vi "Calculator.vi"() -> ()   [LabVIEW 2022 SP3]
uses:
  <vilib>/gmath/NI_Gmath.lvlib
panel:
  in  "%":bool
  in  "pi":bool
  in  "^":bool
  in  "^2":bool
  in  "InputToM1":bool=TRUE
  out "M2":string
  out "M1":string
  in  "M+":bool
  in  "M-":bool
  in  "MR":bool
  in  "MC":bool
  in  "CE":bool
  in  "+/-":bool
  out "Using Time (sec)":dbl
  out "Current Time":timestamp format="%<%Y/%m/%d %H:%M:%S>T"
  in  "power":bool
  out "main":string
  in  "Off":bool
  in  "backspace":bool
  in  "(":bool
  in  ")":bool
  in  "C":bool
  in  "1/x":bool
  in  "Sqrt":bool
  in  "=":bool
  in  "+":bool
  in  "-":bool
  in  "*":bool
  in  "/":bool
  in  "7":bool
  in  "8":bool
  in  "9":bool
  in  "6":bool
  in  "5":bool
  in  "4":bool
  in  "1":bool
  in  "2":bool
  in  "3":bool
  in  ".":bool
  in  "0":bool
  in  "Error":bool
  in  "last_op":u32
  in  "if M":bool
  out "timer_i":dbl
  out "positive":bool=TRUE
  out "answer":dbl
  in  "if\"=\"":bool
  # "Student ID: 111550073"
  # "Guide book:\n\nC : The memories and the screen will be cleared up.\nCE : Only the screen will be cleared up.\n<- : Backspace.\n\n+, -, *, / : When the answer is displayed, you can press then to keep calculate.\n\n1/x : When the string ends with a number, \n         it will input \"(1/\" before the number and a \")\" must be input after you finish inputting.\n         When it ends with an operation symbol, \n         it will input \"(1/\", and a \")\" must be input after you finish inputting.\n         When answer is displayed and it is pressed, you won't have to input a \")\".\n^: Power of. It will input \"^\".\nsqare: It will input \"^2\"\nsqrt : Sqareroot.\n      When the string ends with a number, \n      it will input \"sqrt(\" before the number and a \")\" must be input after you finish inputting.\n      When it ends with an operation symbol, \n      it will input \"sqrt(\", and a \")\" must be input after you finish inputting.\n      When answer is displayed and it is pressed, you won't have to input a \")\".\n£k : pi(x).\n      When the string ends with a number, \n      it will input \"pi(\" before the number and a \")\" must be input after you finish inputting.\n      When it ends with an operation symbol, \n      it will input \"pi(\", and a \")\" must be input after you finish inputting.\n      When answer is displayed and it is pressed, you won't have to input a \")\".\n%: It will input \"*0.01\".\n      When the answer is displayed, you can press then to keep calculate.\n\n+/- : When pressed, it will input a negative symbol before the last number you input.\n          If clicked second time, it will remove the negative symbol.\n          p.s. When the operation symbol is \"-\", it won't change it into a \"+\".\n\nM+, M- : The value on the screen or the answer of the formula will be stored. \nMR : The value which is stored into memory will display on the screen.\nMC : The value in memory will be cleared up. (Either memory 1 or memory 2) \n\nUsing M1& M2: When vertical switch is up, the value will stored into M1; \n                              otherwise, it will be stored into M2."
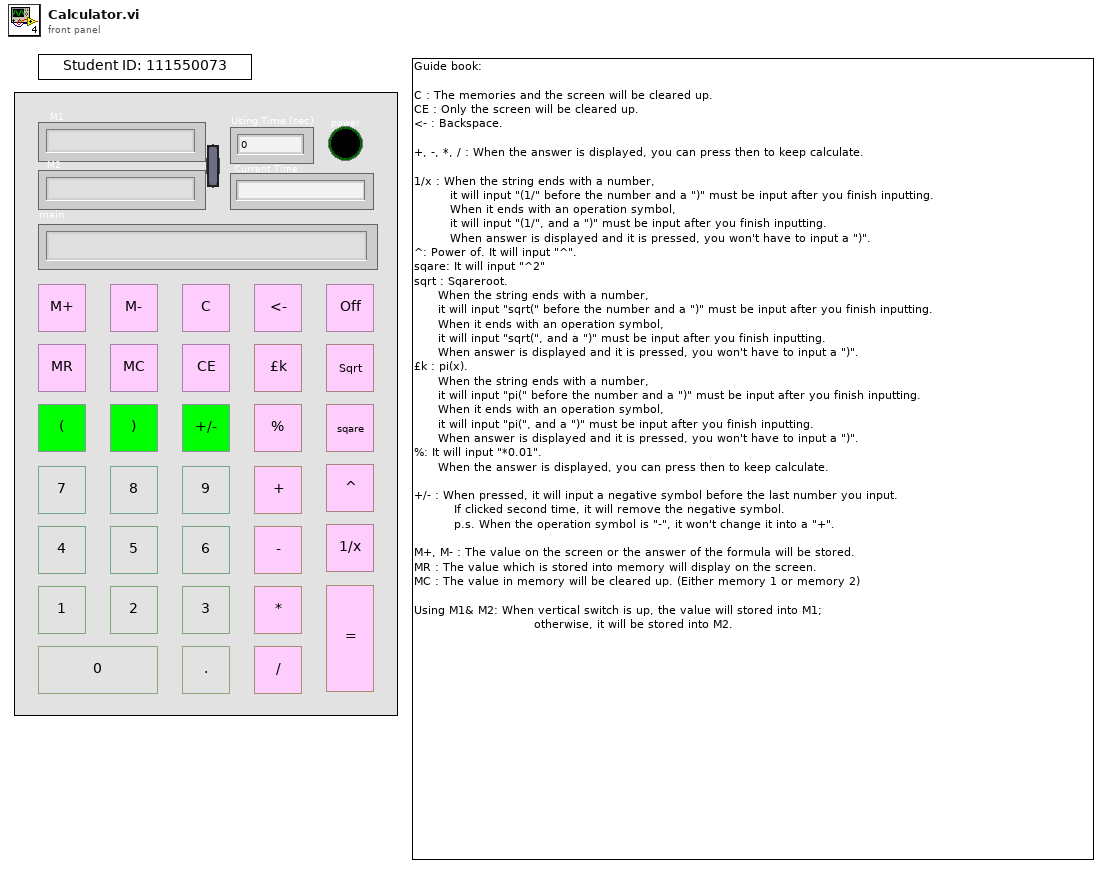
[diagram p1: front panel]
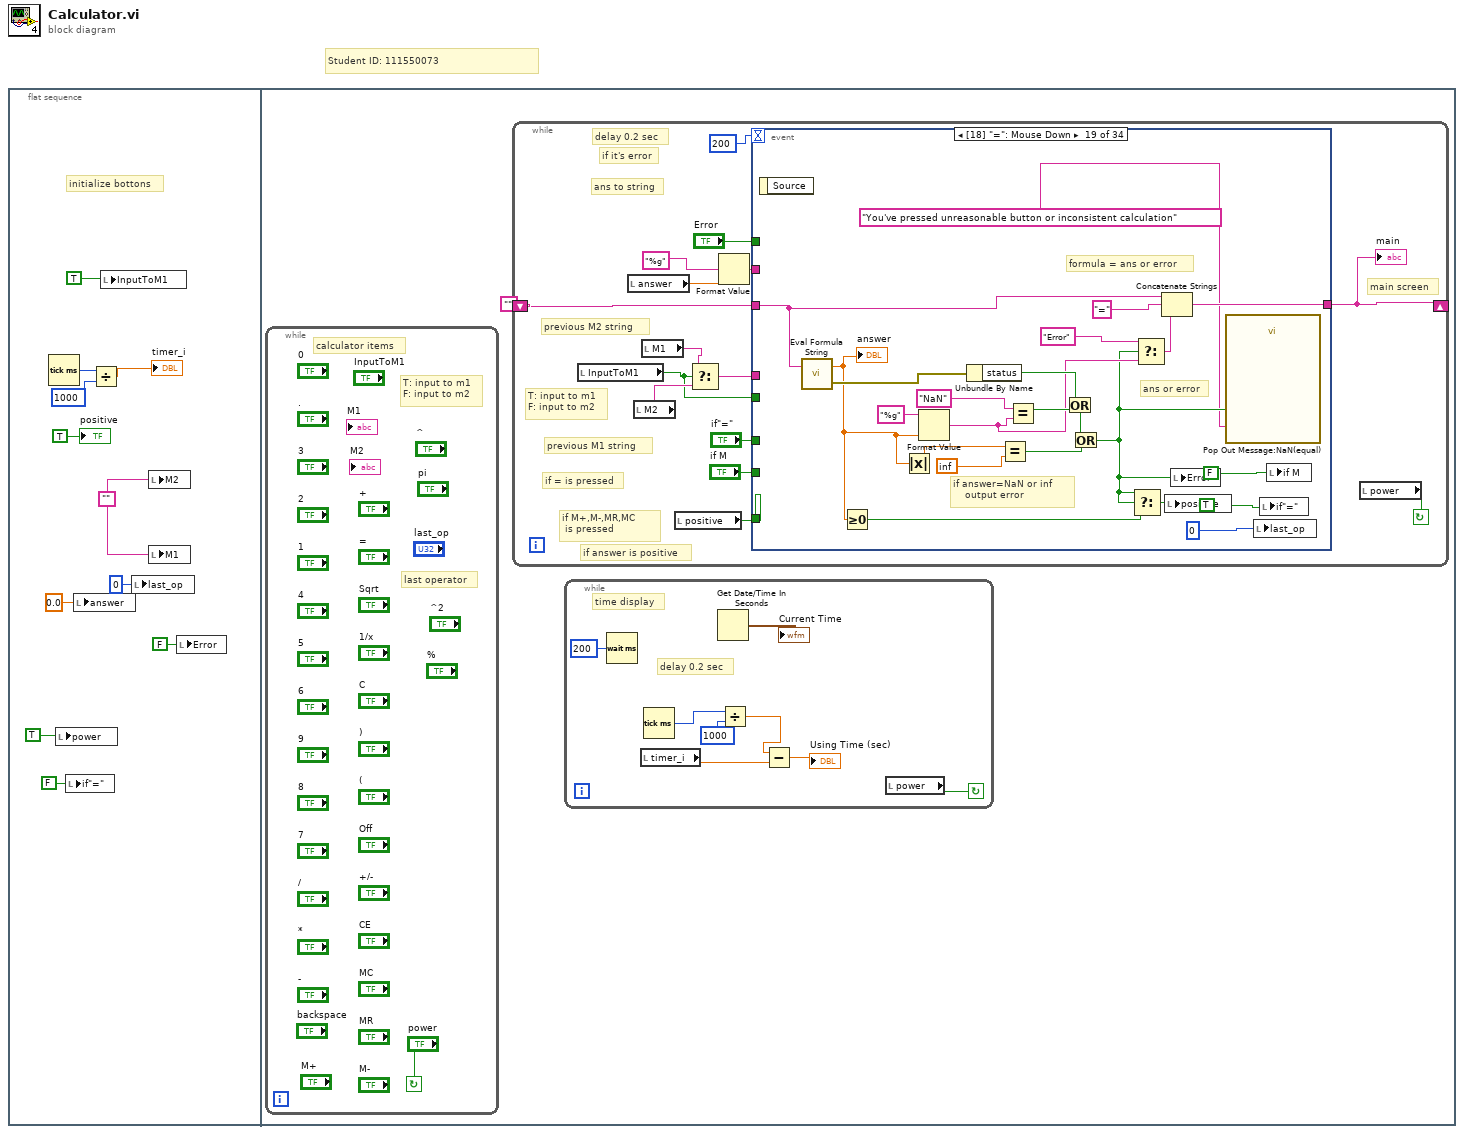
[diagram p0: block diagram]
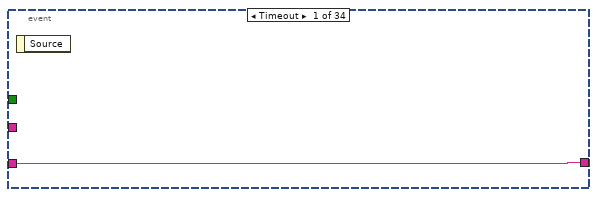
[diagram p2: hidden frame]
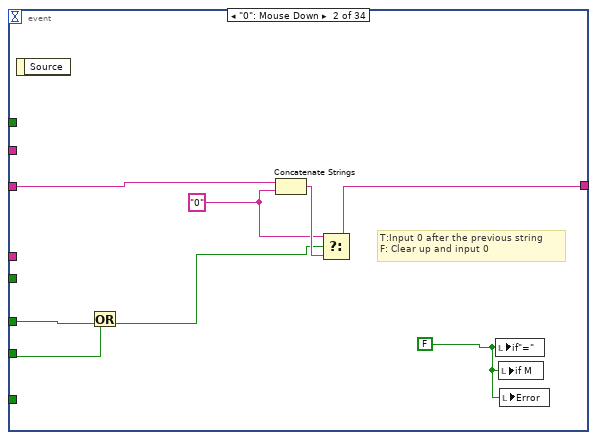
[diagram p3: hidden frame]
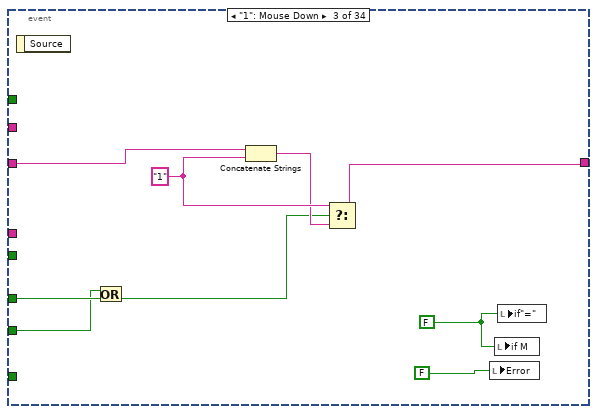
[diagram p4: hidden frame]
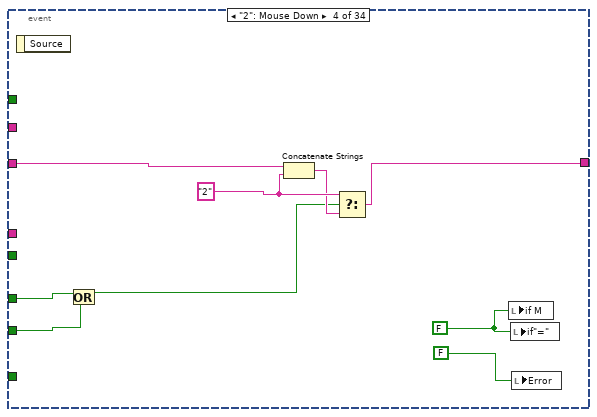
[diagram p5: hidden frame]
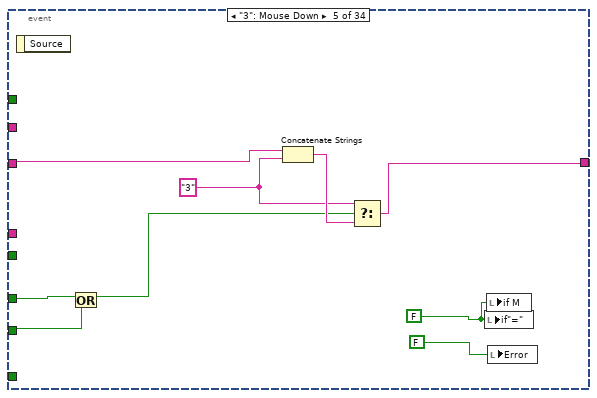
[diagram p6: hidden frame]
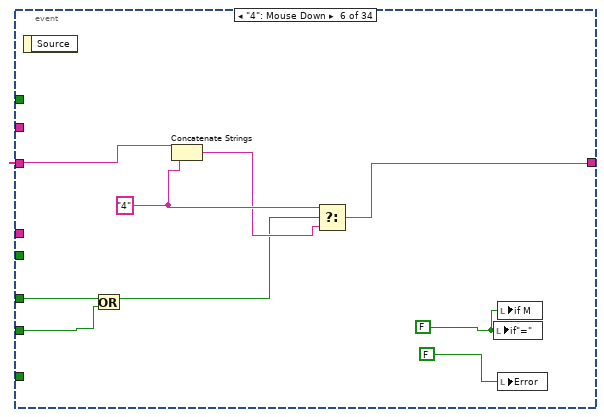
[diagram p7: hidden frame]
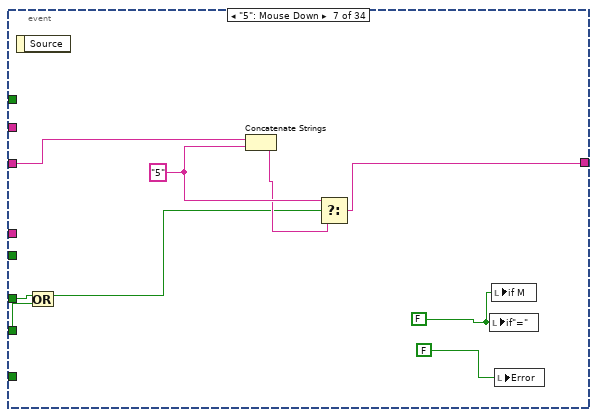
[diagram p8: hidden frame]
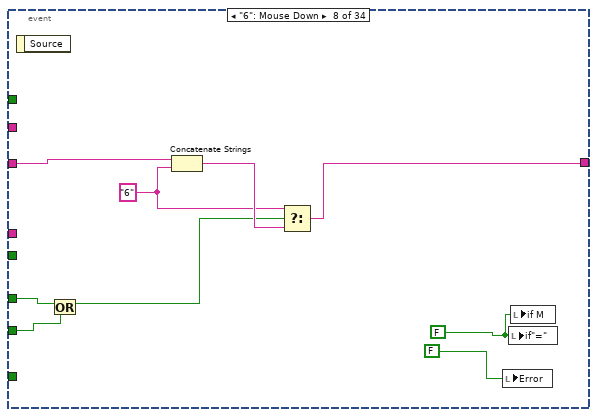
[diagram p9: hidden frame]
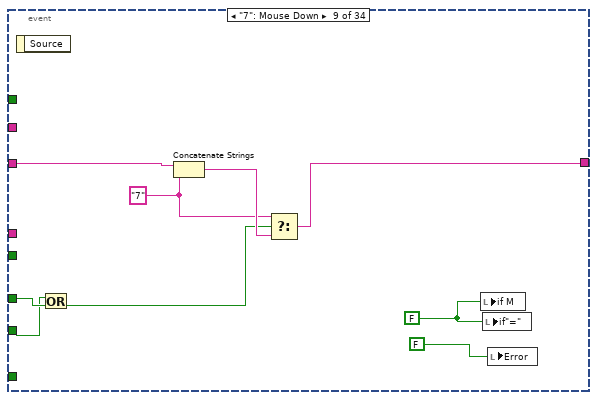
[diagram p10: hidden frame]
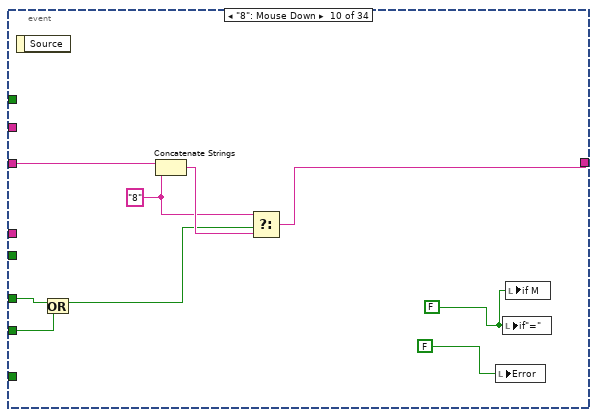
[diagram p11: hidden frame]
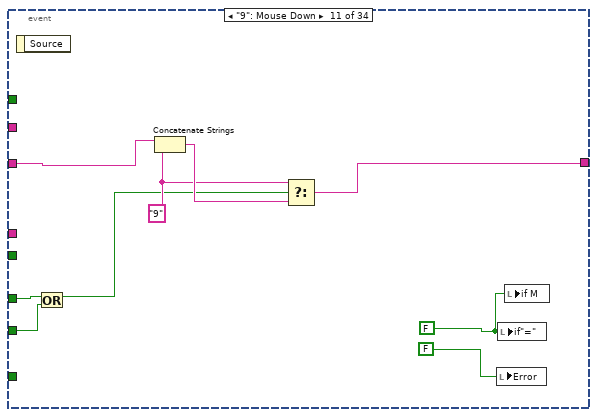
[diagram p12: hidden frame]
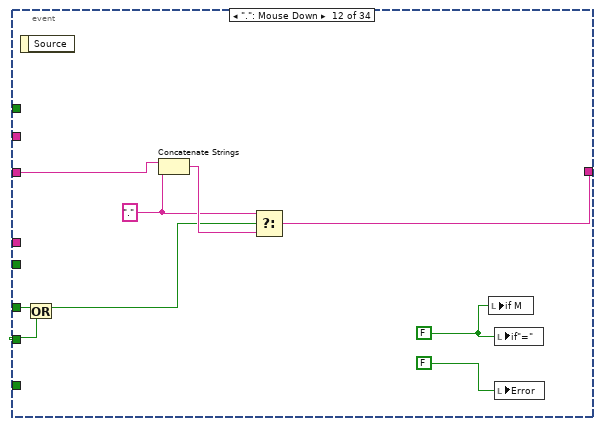
[diagram p13: hidden frame]
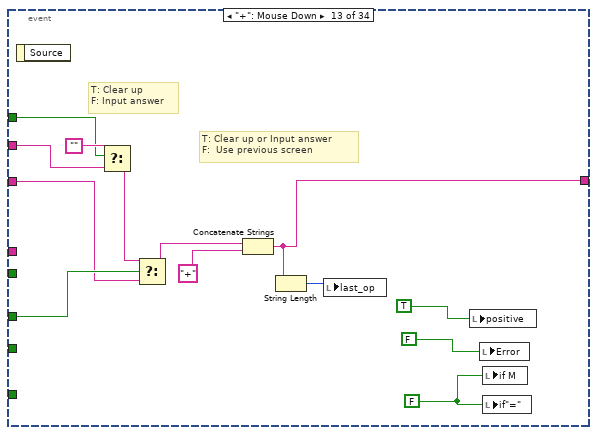
[diagram p14: hidden frame]
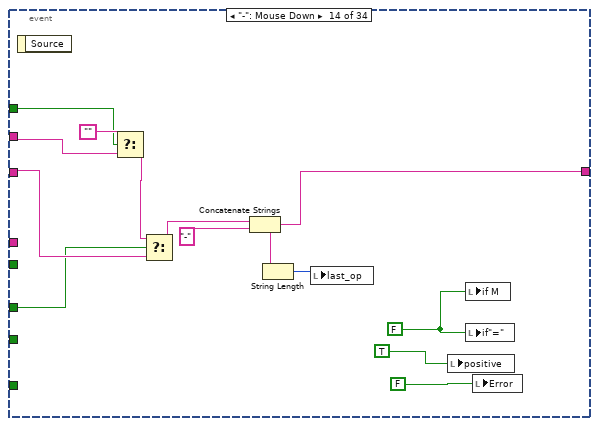
[diagram p15: hidden frame]
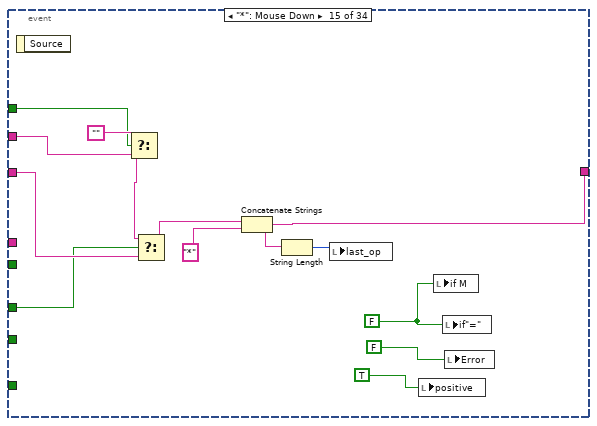
[diagram p16: hidden frame]
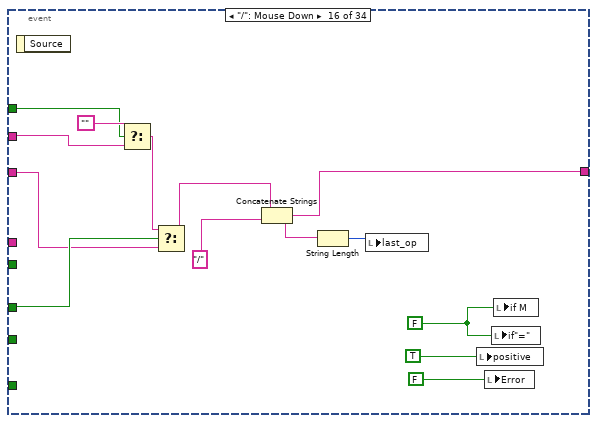
[diagram p17: hidden frame]
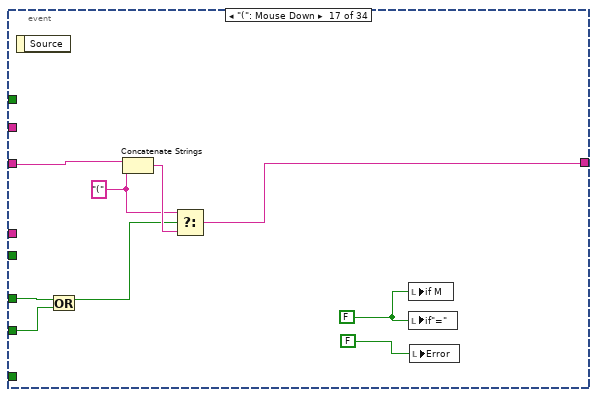
[diagram p18: hidden frame]
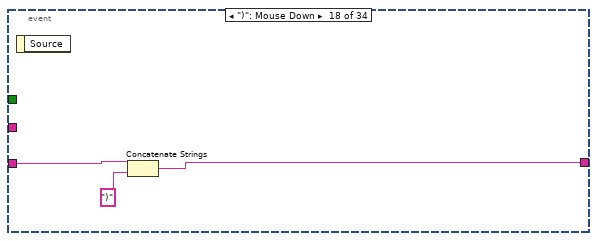
[diagram p19: hidden frame]
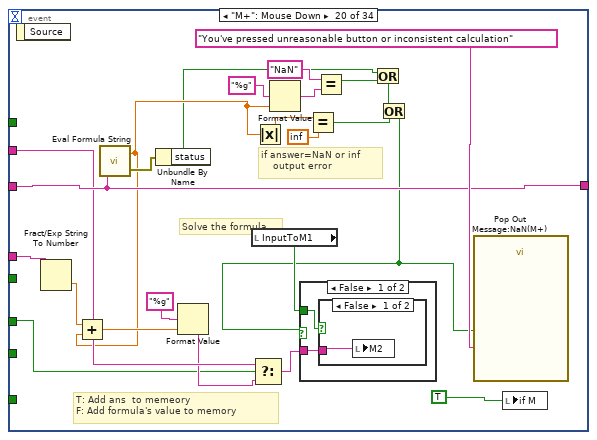
[diagram p20: hidden frame]
diagram:
  # "Student ID: 111550073"
  n1 = flat-sequence {
    frame #0 {
      w3 = ""
      # "initialize bottons"
      n2 = Tick Count (ms)() -> (millisecond timer value=w6:u32)
      n3 = local write "power"(TRUE ("stop")) -> ()
      n4 = local write "if\"=\""(FALSE ("if\"=\"")) -> ()
      n5 = local write "answer"(0.0 ("pre_ans")) -> ()
      n6 = Divide(x=w6, y=u32 1000) -> (x/y=→"timer_i":dbl)
      n7 = local write "InputToM1"(TRUE) -> ()
      n8 = local write "last_op"(u32 0 ("last_op")) -> ()
      n9 = local write "M2"(w3) -> ()
      n10 = local write "M1"(w3) -> ()
      n11 = local write "Error"(FALSE ("Error")) -> ()
      "positive" <- TRUE ("Boolean")
    }
    frame #1 {
      n12 = while {
        stop <- "power" continue-if-true
        # "last operator"
        # "T: input to m1\nF: input to m2"
        # "calculator items"
      }
      n13 = while {
        shift-right: [w33] -> _
        shift-left: "" -> [w21]
        stop <- w24 continue-if-true
        # "delay 0.2 sec"
        # "if it's error"
        # "main screen"
        # "if M+,M-,MR,MC\n is pressed"
        # "if = is pressed"
        # "previous M2 string"
        # "previous M1 string"
        # "T: input to m1\nF: input to m2"
        # "if answer is positive"
        # "ans to string"
        n14 = local read "InputToM1"() -> (w23:bool)
        n15 = local read "answer"() -> (w31:dbl)
        n16 = local read "M2"() -> (w27:string)
        n17 = local read "M1"() -> (w26:string)
        n18 = local read "positive"() -> (w29:bool)
        n19 = Select(t=w26, s=w23, f=w27) -> (s? t:f=w25:string)
        n20 = Format Value(format string="%g", value (0)=w31) -> (output string=w30:string)  [unwired: 1 in]
        n21 = event shown="[18] \"=\": Mouse Down" {
          selector: _ -> [_ _ _ _ _ _ _ _ _ _ _ _ _ _ _ _ _ _ _ _ _ _ _ _ _ _ _ _ _ _ _ _ _ _]
          dyn-events: _ -> [_ _ _ _ _ _ _ _ _ _ _ _ _ _ _ _ _ _ _ _ _ _ _ _ _ _ _ _ _ _ _ _ _ _]
          timeout: 200 -> [_ _ _ _ _ _ _ _ _ _ _ _ _ _ _ _ _ _ _ _ _ _ _ _ _ _ _ _ _ _ _ _ _ _]
          tunnel: [w36 w41 w50 w59 w67 w78 w85 w94 w103 w112 w118 w130 w141 w156 w168 w180 w191 w196 w213 w237 w266 w283 w294 w304 w309 w323 w339 w346 w352 w365 w379 w391 w405 w419] -> w33
          tunnel: w21 -> [w36 w44 w53 w62 w71 w80 w89 w98 w105 w113 w122 w131 w145 w159 w172 w185 w192 w198 w218 w237 w266 w282 w294 w305 w313 w322 w342 w343 w354 w366 w381 w394 w417 w422]
          tunnel: "if\"=\"" -> [_ w42 w51 w60 w68 w79 w86 w95 w104 w114 w123 w132 w146 w149 w162 w186 w193 _ _ w233 w263 w284 _ _ _ w321 _ _ w353 w364 w378 w395 w409 w424]
          tunnel: w29 -> [_ _ _ _ _ _ _ _ _ _ _ _ _ _ _ _ _ _ _ _ _ _ _ _ _ w324 _ _ _ _ _ _ _ _]
          tunnel: w30 -> [_ _ _ _ _ _ _ _ _ _ _ _ w138 w152 w164 w176 _ _ _ w236 w264 _ _ _ _ w315 _ _ w355 w367 w380 w396 w412 w423]
          tunnel: "if M" -> [_ w39 w47 w56 w65 w74 w83 w92 w101 w110 w120 w128 _ _ _ _ w189 _ _ _ _ _ _ _ _ _ _ _ _ _ _ _ _ _]
          tunnel: w25 -> [_ _ _ _ _ _ _ _ _ _ _ _ _ _ _ _ _ _ _ w243 w274 w281 _ _ _ _ _ _ _ _ _ _ _ _]
          tunnel: w23 -> [_ _ _ _ _ _ _ _ _ _ _ _ _ _ _ _ _ _ _ _ _ _ w288 _ _ _ _ _ _ _ _ _ _ _]
          tunnel: "Error" -> [_ _ _ _ _ _ _ _ _ _ _ _ w135 w148 w161 w174 _ _ _ _ _ _ _ _ _ w314 _ _ w349 w368 w382 w397 w406 _]
          event Timeout {
            n22 = event-data() -> ()  [unwired: 1 in, 1 out]
          }
          event "0": Mouse Down {
            w38 = FALSE ("if\"=\"")
            w37 = "0"
            # "T:Input 0 after the previous string\nF: Clear up and input 0"
            n23 = event-data() -> ()  [unwired: 1 in, 1 out]
            n24 = Or(x=w39, y=w42) -> (x .or. y?=w40:bool)
            n25 = Concatenate Strings(w44, w37) -> (w43:string)
            n26 = Select(t=w37, s=w40, f=w43) -> (s? t:f=w41:string)
            n27 = local write "if\"=\""(w38) -> ()
            n28 = local write "if M"(w38) -> ()
            n29 = local write "Error"(w38) -> ()
          }
          event "1": Mouse Down {
            w46 = FALSE ("if\"=\"")
            w52 = "1"
            n30 = event-data() -> ()  [unwired: 1 in, 1 out]
            n31 = Or(x=w47, y=w51) -> (x .or. y?=w48:bool)
            n32 = Concatenate Strings(w53, w52) -> (w49:string)
            n33 = Select(t=w52, s=w48, f=w49) -> (s? t:f=w50:string)
            n34 = local write "Error"(FALSE ("Error")) -> ()
            n35 = local write "if M"(w46) -> ()
            n36 = local write "if\"=\""(w46) -> ()
          }
          event "2": Mouse Down {
            w55 = FALSE ("if\"=\"")
            w61 = "2"
            n37 = event-data() -> ()  [unwired: 1 in, 1 out]
            n38 = Or(x=w60, y=w56) -> (x .or. y?=w57:bool)
            n39 = Concatenate Strings(w62, w61) -> (w58:string)
            n40 = Select(t=w61, s=w57, f=w58) -> (s? t:f=w59:string)
            n41 = local write "if M"(w55) -> ()
            n42 = local write "if\"=\""(w55) -> ()
            n43 = local write "Error"(FALSE ("Error")) -> ()
          }
          event "3": Mouse Down {
            w64 = FALSE ("if\"=\"")
            w69 = "3"
            n44 = event-data() -> ()  [unwired: 1 in, 1 out]
            n45 = Or(x=w68, y=w65) -> (x .or. y?=w66:bool)
            n46 = Concatenate Strings(w71, w69) -> (w70:string)
            n47 = Select(t=w69, s=w66, f=w70) -> (s? t:f=w67:string)
            n48 = local write "if\"=\""(w64) -> ()
            n49 = local write "if M"(w64) -> ()
            n50 = local write "Error"(FALSE ("Error")) -> ()
          }
          event "4": Mouse Down {
            w73 = FALSE ("if\"=\"")
            w77 = "4"
            n51 = event-data() -> ()  [unwired: 1 in, 1 out]
            n52 = Or(x=w79, y=w74) -> (x .or. y?=w75:bool)
            n53 = Concatenate Strings(w80, w77) -> (w76:string)
            n54 = Select(t=w77, s=w75, f=w76) -> (s? t:f=w78:string)
            n55 = local write "if\"=\""(w73) -> ()
            n56 = local write "if M"(w73) -> ()
            n57 = local write "Error"(FALSE ("Error")) -> ()
          }
          event "5": Mouse Down {
            w82 = FALSE ("if\"=\"")
            w88 = "5"
            n58 = event-data() -> ()  [unwired: 1 in, 1 out]
            n59 = Or(x=w86, y=w83) -> (x .or. y?=w84:bool)
            n60 = Concatenate Strings(w89, w88) -> (w87:string)
            n61 = Select(t=w88, s=w84, f=w87) -> (s? t:f=w85:string)
            n62 = local write "if\"=\""(w82) -> ()
            n63 = local write "if M"(w82) -> ()
            n64 = local write "Error"(FALSE ("Error")) -> ()
          }
          event "6": Mouse Down {
            w91 = FALSE ("if\"=\"")
            w96 = "6"
            n65 = event-data() -> ()  [unwired: 1 in, 1 out]
            n66 = Or(x=w95, y=w92) -> (x .or. y?=w93:bool)
            n67 = Concatenate Strings(w98, w96) -> (w97:string)
            n68 = Select(t=w96, s=w93, f=w97) -> (s? t:f=w94:string)
            n69 = local write "Error"(FALSE ("Error")) -> ()
            n70 = local write "if\"=\""(w91) -> ()
            n71 = local write "if M"(w91) -> ()
          }
          event "7": Mouse Down {
            w100 = FALSE ("if\"=\"")
            w106 = "7"
            n72 = event-data() -> ()  [unwired: 1 in, 1 out]
            n73 = Or(x=w101, y=w104) -> (x .or. y?=w102:bool)
            n74 = Concatenate Strings(w105, w106) -> (w107:string)
            n75 = Select(t=w106, s=w102, f=w107) -> (s? t:f=w103:string)
            n76 = local write "if M"(w100) -> ()
            n77 = local write "if\"=\""(w100) -> ()
            n78 = local write "Error"(FALSE ("Error")) -> ()
          }
          event "8": Mouse Down {
            w109 = FALSE ("if\"=\"")
            w115 = "8"
            n79 = event-data() -> ()  [unwired: 1 in, 1 out]
            n80 = Or(x=w114, y=w110) -> (x .or. y?=w111:bool)
            n81 = Concatenate Strings(w113, w115) -> (w116:string)
            n82 = Select(t=w115, s=w111, f=w116) -> (s? t:f=w112:string)
            n83 = local write "Error"(FALSE ("Error")) -> ()
            n84 = local write "if\"=\""(w109) -> ()
            n85 = local write "if M"(w109) -> ()
          }
          event "9": Mouse Down {
            w119 = FALSE ("if\"=\"")
            w124 = "9"
            n86 = event-data() -> ()  [unwired: 1 in, 1 out]
            n87 = Or(x=w123, y=w120) -> (x .or. y?=w121:bool)
            n88 = Concatenate Strings(w122, w124) -> (w125:string)
            n89 = Select(t=w124, s=w121, f=w125) -> (s? t:f=w118:string)
            n90 = local write "Error"(FALSE ("Error")) -> ()
            n91 = local write "if\"=\""(w119) -> ()
            n92 = local write "if M"(w119) -> ()
          }
          event ".": Mouse Down {
            w127 = FALSE ("if\"=\"")
            w133 = "."
            n93 = event-data() -> ()  [unwired: 1 in, 1 out]
            n94 = Or(x=w132, y=w128) -> (x .or. y?=w129:bool)
            n95 = Concatenate Strings(w131, w133) -> (w134:string)
            n96 = Select(t=w133, s=w129, f=w134) -> (s? t:f=w130:string)
            n97 = local write "if M"(w127) -> ()
            n98 = local write "if\"=\""(w127) -> ()
            n99 = local write "Error"(FALSE ("Error")) -> ()
          }
          event "+": Mouse Down {
            w144 = FALSE ("if\"=\"")
            # "T: Clear up or Input answer  \nF:  Use previous screen"
            # "T: Clear up\nF: Input answer"
            n100 = event-data() -> ()  [unwired: 1 in, 1 out]
            n101 = Select(t="", s=w135, f=w138) -> (s? t:f=w139:string)
            n102 = Select(t=w139, s=w146, f=w145) -> (s? t:f=w147:string)
            n103 = Concatenate Strings(w147, "+") -> (w141:string)
            n104 = String Length(string=w141) -> (length=w142:i32)
            n105 = local write "last_op"(w142) -> ()
            n106 = local write "positive"(TRUE ("positive")) -> ()
            n107 = local write "Error"(FALSE ("Error")) -> ()
            n108 = local write "if M"(w144) -> ()
            n109 = local write "if\"=\""(w144) -> ()
          }
          event "-": Mouse Down {
            w158 = FALSE ("if\"=\"")
            n110 = event-data() -> ()  [unwired: 1 in, 1 out]
            n111 = Select(t="", s=w148, f=w152) -> (s? t:f=w151:string)
            n112 = Select(t=w151, s=w149, f=w159) -> (s? t:f=w160:string)
            n113 = Concatenate Strings(w160, "-") -> (w156:string)
            n114 = String Length(string=w156) -> (length=w155:i32)
            n115 = local write "last_op"(w155) -> ()
            n116 = local write "positive"(TRUE ("positive")) -> ()
            n117 = local write "if M"(w158) -> ()
            n118 = local write "if\"=\""(w158) -> ()
            n119 = local write "Error"(FALSE ("Error")) -> ()
          }
          event "*": Mouse Down {
            w171 = FALSE ("if\"=\"")
            n120 = event-data() -> ()  [unwired: 1 in, 1 out]
            n121 = Select(t="", s=w161, f=w164) -> (s? t:f=w163:string)
            n122 = Select(t=w163, s=w162, f=w172) -> (s? t:f=w173:string)
            n123 = Concatenate Strings(w173, "*") -> (w168:string)
            n124 = String Length(string=w168) -> (length=w169:i32)
            n125 = local write "last_op"(w169) -> ()
            n126 = local write "positive"(TRUE ("positive")) -> ()
            n127 = local write "if M"(w171) -> ()
            n128 = local write "if\"=\""(w171) -> ()
            n129 = local write "Error"(FALSE ("Error")) -> ()
          }
          event "/": Mouse Down {
            w183 = FALSE ("if\"=\"")
            n130 = event-data() -> ()  [unwired: 1 in, 1 out]
            n131 = Select(t="", s=w174, f=w176) -> (s? t:f=w175:string)
            n132 = Select(t=w175, s=w186, f=w185) -> (s? t:f=w184:string)
            n133 = Concatenate Strings(w184, "/") -> (w180:string)
            n134 = String Length(string=w180) -> (length=w181:i32)
            n135 = local write "last_op"(w181) -> ()
            n136 = local write "positive"(TRUE ("positive")) -> ()
            n137 = local write "Error"(FALSE ("Error")) -> ()
            n138 = local write "if\"=\""(w183) -> ()
            n139 = local write "if M"(w183) -> ()
          }
          event "(": Mouse Down {
            w188 = FALSE ("if\"=\"")
            w194 = "("
            n140 = event-data() -> ()  [unwired: 1 in, 1 out]
            n141 = Or(x=w193, y=w189) -> (x .or. y?=w190:bool)
            n142 = Concatenate Strings(w192, w194) -> (w195:string)
            n143 = Select(t=w194, s=w190, f=w195) -> (s? t:f=w191:string)
            n144 = local write "if M"(w188) -> ()
            n145 = local write "if\"=\""(w188) -> ()
            n146 = local write "Error"(FALSE ("Error")) -> ()
          }
          event ")": Mouse Down {
            n147 = event-data() -> ()  [unwired: 1 in, 1 out]
            n148 = Concatenate Strings(w198, ")") -> (w196:string)
          }
          event "=": Mouse Down {
            # "if answer=NaN or inf \n    output error"
            # "ans or error"
            # "formula = ans or error"
            n149 = event-data() -> ()  [unwired: 1 in, 1 out]
            n150 = call <vilib>:"Eval Formula String.vi"("formula"=w218) -> ("error out"=w216:errorcluster, "y value"=w199:dbl)  [unwired: 1 in]
            "answer" <- w199
            n151 = Greater Or Equal To 0?(x=w199) -> (x >= 0?=w204:bool)
            n152 = Absolute Value(x=w199) -> (abs(x)=w212:dbl)
            n153 = Format Value(format string="%g", value (0)=w199) -> (output string=w205:string)  [unwired: 1 in]
            n154 = Unbundle By Name(w216) -> ("status"=w208:bool)
            n155 = Equal?(x=w212, y=inf) -> (x = y?=w210:bool)
            n156 = Equal?(x="NaN", y=w205) -> (x = y?=w206:bool)
            n157 = Or(x=w208, y=w206) -> (x .or. y?=w207:bool)
            n158 = Or(x=w207, y=w210) -> (x .or. y?=w201:bool)
            n159 = Select(t=w201, s=w201, f=w204) -> (s? t:f=w203:bool)
            n160 = Select(t="Error" ("f"), s=w201, f=w205) -> (s? t:f=w214:string)
            n161 = Concatenate Strings(w218, "=" ("string"), w214) -> (w213:string)
            n162 = local write "positive"(w203) -> ()
            n163 = local write "Error"(w201) -> ()
            n164 = call "Pop Out Message:NaN(equal)"("Enable"=w201, "Message"="You've pressed unreasonable button or inconsistent calculation") -> ()  [unwired: 8 in, 2 out]
            n165 = local write "last_op"(u32 0 ("last_op")) -> ()
            n166 = local write "if\"=\""(TRUE ("if\"=\"")) -> ()
            n167 = local write "if M"(FALSE ("if\"=\"")) -> ()
          }
          event "M+": Mouse Down {
            # "if answer=NaN or inf \n    output error"
            # "Solve the formula"
            # "T: Add ans  to memeory\nF: Add formula's value to memory"
            n168 = event-data() -> ()  [unwired: 1 in, 1 out]
            n169 = Fract/Exp String To Number(string=w243) -> (number=w242:dbl)  [unwired: 3 in, 1 out]
            n170 = call <vilib>:"Eval Formula String.vi"("formula"=w237) -> ("error out"=w239:errorcluster, "y value"=w224:dbl)  [unwired: 1 in]
            n171 = Add(x=w242, y=w224) -> (x+y=w244:dbl)
            n172 = Unbundle By Name(w239) -> ("status"=w223:bool)
            n173 = Format Value(format string="%g", value (0)=w244) -> (output string=w235:string)  [unwired: 1 in]
            n174 = local read "InputToM1"() -> (w238:bool)
            n175 = Select(t=w236, s=w233, f=w235) -> (s? t:f=w234:string)
            n176 = Absolute Value(x=w224) -> (abs(x)=w232:dbl)
            n177 = Format Value(format string="%g", value (0)=w224) -> (output string=w228:string)  [unwired: 1 in]
            n178 = Equal?(x=w232, y=inf) -> (x = y?=w231:bool)
            n179 = Equal?(x="NaN", y=w228) -> (x = y?=w229:bool)
            n180 = Or(x=w223, y=w229) -> (x .or. y?=w230:bool)
            n181 = Or(x=w230, y=w231) -> (x .or. y?=w222:bool)
            n182 = case shown="False" w222 {
              tunnel: w238 -> [w247 _]
              tunnel: w234 -> [w246 _]
              frame False {
                n183 = case shown="False" w247 {
                  tunnel: w246 -> [w248 w249]
                  frame False {
                    n184 = local write "M2"(w248) -> ()
                  }
                  frame True {
                    n185 = local write "M1"(w249) -> ()
                  }
                }
              }
              frame True {
              }
            }
            n186 = call "Pop Out Message:NaN(M+)"("Enable"=w222, "Message"="You've pressed unreasonable button or inconsistent calculation") -> ()  [unwired: 8 in, 2 out]
            n187 = local write "if M"(TRUE ("if\"=\"")) -> ()
          }
          event "M-": Mouse Down {
            # "if answer=NaN or inf \n    output error"
            # "string to float"
            # "T: Add  negative ans  to memeory\nF: Add formula's negative value to     memory"
            n188 = event-data() -> ()  [unwired: 1 in, 1 out]
            n189 = call <vilib>:"Eval Formula String.vi"("formula"=w266) -> ("error out"=w271:errorcluster, "y value"=w252:dbl)  [unwired: 1 in]
            n190 = Fract/Exp String To Number(string=w274) -> (number=w273:dbl)  [unwired: 3 in, 1 out]
            n191 = Unbundle By Name(w271) -> ("status"=w251:bool)
            n192 = Absolute Value(x=w252) -> (abs(x)=w256:dbl)
            n193 = Format Value(format string="%g", value (0)=w252) -> (output string=w260:string)  [unwired: 1 in]
            n194 = Equal?(x=w256, y=inf) -> (x = y?=w257:bool)
            n195 = Equal?(x="NaN", y=w260) -> (x = y?=w259:bool)
            n196 = Or(x=w251, y=w259) -> (x .or. y?=w258:bool)
            n197 = Or(x=w258, y=w257) -> (x .or. y?=w250:bool)
            n198 = Select(t=0.0, s=w250, f=w252) -> (s? t:f=w268:dbl)
            n199 = Negate(x=w268) -> (-x=w276:dbl)
            n200 = Add(x=w273, y=w276) -> (x+y=w261:dbl)
            n201 = Format Value(format string="%g", value (0)=w261) -> (output string=w265:string)  [unwired: 1 in]
            n202 = Select(t=w264, s=w263, f=w265) -> (s? t:f=w262:string)
            n203 = local read "InputToM1"() -> (w267:bool)
            n204 = case shown="False" w250 {
              tunnel: w267 -> [w278 _]
              tunnel: w262 -> [w277 _]
              frame False {
                n205 = case shown="False" w278 {
                  tunnel: w277 -> [w279 w280]
                  frame False {
                    n206 = local write "M2"(w279) -> ()
                  }
                  frame True {
                    n207 = local write "M1"(w280) -> ()
                  }
                }
              }
              frame True {
              }
            }
            n208 = call "Display Message to User3"("Enable"=w250, "Message"="You've pressed unreasonable button or inconsistent calculation") -> ()  [unwired: 8 in, 2 out]
            n209 = local write "if M"(TRUE ("if\"=\"")) -> ()
          }
          event "MR": Mouse Down {
            # "T:Input memory after the previous string\nF: Clear up and input memory"
            n210 = event-data() -> ()  [unwired: 1 in, 1 out]
            n211 = Concatenate Strings(w282, w281) -> (w285:string)
            n212 = Select(t=w281, s=w284, f=w285) -> (s? t:f=w283:string)
            n213 = local write "if M"(TRUE ("if\"=\"")) -> ()
          }
          event "MC": Mouse Down {
            n214 = event-data() -> ()  [unwired: 1 in, 1 out]
            n215 = Select(t="2?", s=w288, f="1?" ("Message")) -> (s? t:f=w290:string)
            n216 = Concatenate Strings("Are you sure to clear up M" ("Message"), w290) -> (w292:string)
            n217 = call "Pop Out Message:MC"("Message"=w292) -> ("Yes"=w293:bool)  [unwired: 9 in, 1 out]
            n218 = case shown="True" w293 {
              frame False {
              }
              frame True {
                n219 = local read "InputToM1"() -> (w296:bool)
                n220 = case shown="False" w296 {
                  tunnel: "" -> [w297 w298]
                  frame False {
                    n221 = local write "M2"(w297) -> ()
                  }
                  frame True {
                    n222 = local write "M1"(w298) -> ()
                  }
                }
              }
            }
          }
          event "C": Mouse Down {
            n223 = event-data() -> ()  [unwired: 1 in, 1 out]
            n224 = Concatenate Strings("Are you sure to clear up " ("Message"), "the screen and memory?" ("string")) -> (w301:string)
            n225 = call "Pop Out Message:C"("Message"=w301) -> ("Yes"=w300:bool)  [unwired: 9 in, 1 out]
            n226 = case shown="True" w300 {
              frame False {
              }
              frame True {
                w307 = ""
                n227 = local write "M1"(w307) -> ()
                n228 = local write "M2"(w307) -> ()
              }
            }
            n229 = Select(t="", s=w300, f=w305) -> (s? t:f=w304:string)
            n230 = local write "Error"(FALSE ("Error")) -> ()
          }
          event "CE": Mouse Down {
            n231 = event-data() -> ()  [unwired: 1 in, 1 out]
            n232 = call "Pop Out Message:CE"("Message"="Are you sure to clear up the screen?") -> ("Yes"=w311:bool)  [unwired: 9 in, 1 out]
            n233 = Select(t="", s=w311, f=w313) -> (s? t:f=w309:string)
            n234 = local write "Error"(FALSE ("Error")) -> ()
          }
          event "+/-": Mouse Down {
            n235 = event-data() -> ()  [unwired: 1 in, 1 out]
            n236 = Select(t="", s=w314, f=w315) -> (s? t:f=w316:string)
            n237 = Select(t=w316, s=w321, f=w322) -> (s? t:f=w317:string)
            n238 = case shown="True" w324 {
              tunnel: w317 -> [w330 w337]
              tunnel: [w327 w335] -> w323
              frame False {
                n239 = local read "last_op"() -> (w328:u32)
                n240 = local write "positive"(TRUE ("positive")) -> ()
                n241 = Increment(x=w328) -> (x+1=w329:u32)
                n242 = String Subset(string=w330, length (rest)=w328) -> (substring=w326:string)  [unwired: 1 in]
                n243 = String Subset(string=w330, offset (0)=w329) -> (substring=w325:string)  [unwired: 1 in]
                n244 = Concatenate Strings(w326, w325) -> (w327:string)
              }
              frame True {
                n245 = local read "last_op"() -> (w336:u32)
                n246 = local write "positive"(FALSE ("positive")) -> ()
                n247 = String Subset(string=w337, length (rest)=w336) -> (substring=w333:string)  [unwired: 1 in]
                n248 = String Subset(string=w337, offset (0)=w336) -> (substring=w332:string)  [unwired: 1 in]
                n249 = Concatenate Strings(w333, "-" ("string"), w332) -> (w335:string)
              }
            }
            n250 = local write "Error"(FALSE ("Error")) -> ()
            n251 = local write "if\"=\""(FALSE ("if\"=\"")) -> ()
          }
          event "backspace": Mouse Down {
            n252 = event-data() -> ()  [unwired: 1 in, 1 out]
            n253 = String Length(string=w342) -> (length=w341:i32)
            n254 = Decrement(x=w341) -> (x-1=w340:i32)
            n255 = String Subset(string=w342, length (rest)=w340) -> (substring=w339:string)  [unwired: 1 in]
          }
          event "Off": Mouse Down {
            n256 = event-data() -> ()  [unwired: 1 in, 1 out]
            n257 = call "Pop Out Message:Calculator Off"("Message"="Are you sure to turn off?") -> ("Yes"=w344:bool)  [unwired: 9 in, 1 out]
            n258 = Not(x=w344) -> (.not. x?=w345:bool)
            n259 = local write "power"(w345) -> ()
            n260 = Select(t="", s=w344, f=w343) -> (s? t:f=w346:string)
          }
          event "Sqrt": Mouse Down {
            w350 = "sqrt(" ("string")
            n261 = event-data() -> ()  [unwired: 1 in, 1 out]
            n262 = local read "last_op"() -> (w359:u32)
            n263 = String Subset(string=w354, length (rest)=w359) -> (substring=w360:string)  [unwired: 1 in]
            n264 = String Subset(string=w354, offset (0)=w359) -> (substring=w361:string)  [unwired: 1 in]
            n265 = Concatenate Strings(w350, w355, ")" ("string")) -> (w356:string)
            n266 = Concatenate Strings(w360, w350, w361) -> (w358:string)
            n267 = Select(t=w356, s=w353, f=w358) -> (s? t:f=w351:string)
            n268 = Select(t=w350, s=w349, f=w351) -> (s? t:f=w352:string)
            n269 = local write "Error"(FALSE ("Error")) -> ()
            n270 = local write "if\"=\""(FALSE ("if\"=\"")) -> ()
          }
          event "1/x": Mouse Down {
            w370 = "(1/" ("string")
            n271 = event-data() -> ()  [unwired: 1 in, 1 out]
            n272 = local read "last_op"() -> (w374:u32)
            n273 = String Subset(string=w366, length (rest)=w374) -> (substring=w375:string)  [unwired: 1 in]
            n274 = String Subset(string=w366, offset (0)=w374) -> (substring=w376:string)  [unwired: 1 in]
            n275 = Concatenate Strings(w370, w367, ")" ("string")) -> (w372:string)
            n276 = Concatenate Strings(w375, w370, w376) -> (w373:string)
            n277 = Select(t=w372, s=w364, f=w373) -> (s? t:f=w371:string)
            n278 = Select(t=w370, s=w368, f=w371) -> (s? t:f=w365:string)
            n279 = local write "Error"(FALSE ("Error")) -> ()
          }
          event "^": Mouse Down {
            w389 = FALSE ("if\"=\"")
            # "T: Clear up or Input answer  \nF:  Use previous screen"
            # "T: Clear up\nF: Input answer"
            n280 = event-data() -> ()  [unwired: 1 in, 1 out]
            n281 = Select(t="", s=w382, f=w380) -> (s? t:f=w385:string)
            n282 = Select(t=w385, s=w378, f=w381) -> (s? t:f=w390:string)
            n283 = Concatenate Strings(w390, "^") -> (w379:string)
            n284 = String Length(string=w379) -> (length=w387:i32)
            n285 = local write "last_op"(w387) -> ()
            n286 = local write "positive"(TRUE ("positive")) -> ()
            n287 = local write "Error"(FALSE ("Error")) -> ()
            n288 = local write "if M"(w389) -> ()
            n289 = local write "if\"=\""(w389) -> ()
          }
          event "^2": Mouse Down {
            w398 = FALSE ("if\"=\"")
            # "T: Clear up or Input answer  \nF:  Use previous screen"
            # "T: Clear up\nF: Input answer"
            n290 = event-data() -> ()  [unwired: 1 in, 1 out]
            n291 = Select(t="", s=w397, f=w396) -> (s? t:f=w402:string)
            n292 = Select(t=w402, s=w395, f=w394) -> (s? t:f=w404:string)
            n293 = Concatenate Strings(w404, "^2" ("string")) -> (w391:string)
            n294 = String Length(string=w391) -> (length=w403:i32)
            n295 = Decrement(x=w403) -> (x-1=w392:i32)
            n296 = local write "last_op"(w392) -> ()
            n297 = local write "positive"(TRUE ("positive")) -> ()
            n298 = local write "Error"(FALSE ("Error")) -> ()
            n299 = local write "if M"(w398) -> ()
            n300 = local write "if\"=\""(w398) -> ()
          }
          event "pi": Mouse Down {
            w414 = FALSE ("if\"=\"")
            w407 = "pi(" ("string")
            n301 = event-data() -> ()  [unwired: 1 in, 1 out]
            n302 = local read "last_op"() -> (w415:u32)
            n303 = String Subset(string=w417, length (rest)=w415) -> (substring=w416:string)  [unwired: 1 in]
            n304 = String Subset(string=w417, offset (0)=w415) -> (substring=w418:string)  [unwired: 1 in]
            n305 = Concatenate Strings(w407, w412, ")" ("string")) -> (w410:string)
            n306 = Concatenate Strings(w416, w407, w418) -> (w413:string)
            n307 = Select(t=w410, s=w409, f=w413) -> (s? t:f=w408:string)
            n308 = Select(t=w407, s=w406, f=w408) -> (s? t:f=w405:string)
            n309 = local write "if\"=\""(w414) -> ()
            n310 = local write "if M"(w414) -> ()
            n311 = local write "Error"(w414) -> ()
          }
          event "%": Mouse Down {
            w425 = FALSE ("if\"=\"")
            # "T:Input *0.01 after the previous string\nF: Clear up and input ans*0.01"
            n312 = event-data() -> ()  [unwired: 1 in, 1 out]
            n313 = Select(t=w423, s=w424, f=w422) -> (s? t:f=w421:string)
            n314 = Concatenate Strings(w421, "*0.01" ("string")) -> (w419:string)
            n315 = local write "if\"=\""(w425) -> ()
            n316 = local write "if M"(w425) -> ()
          }
        }
        "main" <- w33
        n317 = local read "power"() -> (w24:bool)
      }
      n318 = while {
        stop <- w17 continue-if-true
        # "delay 0.2 sec"
        # "time display"
        n319 = Wait (ms)(milliseconds to wait=u32 200) -> ()  [unwired: 1 out]
        n320 = local read "timer_i"() -> (w20:dbl)
        n321 = Tick Count (ms)() -> (millisecond timer value=w15:u32)
        n322 = Get Date/Time In Seconds() -> (seconds since 1Jan1904=→"Current Time":timestamp)
        n323 = Divide(x=w15, y=u32 1000) -> (x/y=w13:dbl)
        n324 = Subtract(x=w13, y=w20) -> (x-y=→"Using Time (sec)":dbl)
        n325 = local read "power"() -> (w17:bool)
      }
    }
  }
